vi "Set w4lvgrpc_ToServer.vi"(7 "Complete Call (T)":bool=TRUE, 8 "error in (no error)":errorcluster, 10 "package_templatemessage":T1, 11 "gRPCid":T2) -> (0 "error out":errorcluster)   [LabVIEW 2019, in "Generated_server.lvlib"]
uses:
  Generated_server.lvlib
  <vilib>/gRPC/LabVIEW gRPC Library/grpc-lvsupport-release.lvlib
  dcc74a39-081a-4bdd-860b-8ed792803c96.vi
  w4lvgrpc_Msg_ToServer_1_Flat.ctl
  w4lvgrpc_Msg_ToServer_2_Flat.ctl
  w4lvgrpc_Msg_ToServer_3_Flat.ctl
  w4lvgrpc_Msg_ToServer_4_Flat.ctl
  w4lvgrpc_Msg_ToServer_5_Flat.ctl
  w4lvgrpc_Msg_ToServer_6_Flat.ctl
  w4lvgrpc_Msg_ToServer_7_Flat.ctl
  w4lvgrpc_Msg_ToServer_8_Flat.ctl
  w4lvgrpc_Msg_ToServer_9_Flat.ctl
  w4lvgrpc_ToServer_Flat.ctl
  <vilib>/gRPC/LabVIEW gRPC Library/Shared/grpcId.ctl
  w4lvgrpc_ToServer_payload/w4lvgrpc_ToServer_payload.lvclass
  w4lvgrpc_ToServer.ctl
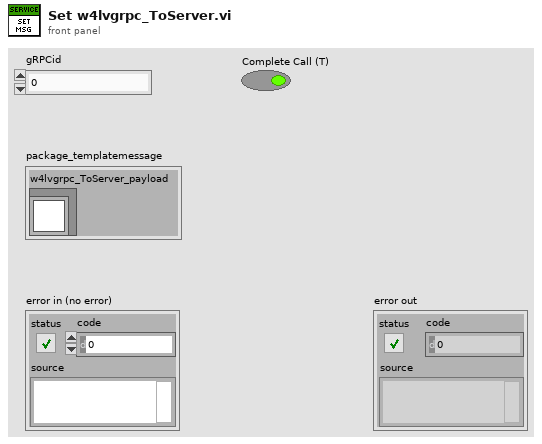
[diagram p1: front panel]
types:
  T1 = typedef "Generated_server.lvlib/w4lvgrpc_ToServer.ctl" = cluster{"w4lvgrpc_ToServer_payload":refnum<class "w4lvgrpc_ToServer_payload.lvclass">}
  T2 = typedef "grpc-lvsupport-release.lvlib/grpcId.ctl" = u64
  T3 = typedef "Generated_server.lvlib/w4lvgrpc_ToServer_Flat.ctl" = cluster{"w4lvgrpc_ToServer_payload_selected_index":i32, "msg_1":T4, "msg_2":T5, "msg_3":T6, "msg_4":T7, "msg_5":T8, "msg_6":T9, "msg_7":T10, "msg_8":T11, "msg_9":T12}
  T4 = typedef "Generated_server.lvlib/w4lvgrpc_Msg_ToServer_1_Flat.ctl" = cluster{"placeholder":string}
  T5 = typedef "Generated_server.lvlib/w4lvgrpc_Msg_ToServer_2_Flat.ctl" = cluster{"placeholder":string}
  T6 = typedef "Generated_server.lvlib/w4lvgrpc_Msg_ToServer_3_Flat.ctl" = cluster{"placeholder":string}
  T7 = typedef "Generated_server.lvlib/w4lvgrpc_Msg_ToServer_4_Flat.ctl" = cluster{"placeholder":string}
  T8 = typedef "Generated_server.lvlib/w4lvgrpc_Msg_ToServer_5_Flat.ctl" = cluster{"placeholder":string}
  T9 = typedef "Generated_server.lvlib/w4lvgrpc_Msg_ToServer_6_Flat.ctl" = cluster{"placeholder":string}
  T10 = typedef "Generated_server.lvlib/w4lvgrpc_Msg_ToServer_7_Flat.ctl" = cluster{"placeholder":string}
  T11 = typedef "Generated_server.lvlib/w4lvgrpc_Msg_ToServer_8_Flat.ctl" = cluster{"placeholder":string}
  T12 = typedef "Generated_server.lvlib/w4lvgrpc_Msg_ToServer_9_Flat.ctl" = cluster{"placeholder":string}
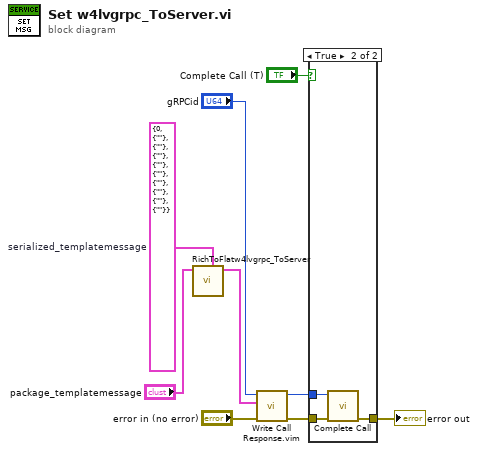
[diagram p0: block diagram]
diagram:
  w2 = T3 {"w4lvgrpc_ToServer_payload_selected_index"=0, "msg_1"={"placeholder"=""}, "msg_2"={"placeholder"=""}, "msg_3"={"placeholder"=""}, "msg_4"={"placeholder"=""}, "msg_5"={"placeholder"=""}, "msg_6"={"placeholder"=""}, "msg_7"={"placeholder"=""}, "msg_8"={"placeholder"=""}, "msg_9"={"placeholder"=""}}  # serialized_templatemessage
  n1 = call "RichToFlatw4lvgrpc_ToServer.vi"("OutputClusterType"=w2, "InputCluster"="package_templatemessage") -> ("OutputCluster"=w1:T3)  [unwired: 9 in]
  n2 = call "Write Call Response.vim"("error in"="error in (no error)", "Response Data"=w1, "gRPCid in"="gRPCid") -> ("error out"=w6:errorcluster, "gRPCid out"=w7:T2)  [unwired: 7 in]
  n3 = case shown="True" "Complete Call (T)" {
    tunnel: [w10 w13] -> w9
    tunnel: w7 -> [_ w12]
    tunnel: w6 -> [w10 w11]
    frame False {
    }
    frame True {
      n4 = call <vilib>:"Complete Call.vi"("gRPCid"=w12, "error in"=w11) -> ("error out"=w13:errorcluster)  [unwired: 8 in]
    }
  }
  "error out" <- w9
